vi "14.vi"(11 "n_Collatz":u64 min=1 step=1) -> (3 "max index(es)":i32)   [LabVIEW 2021]
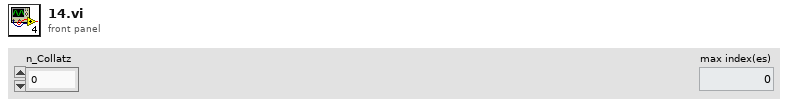
[diagram p1: front panel]
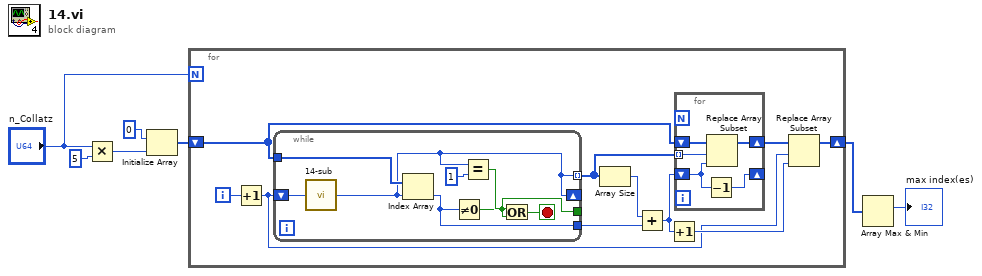
[diagram p0: block diagram]
diagram:
  n1 = Multiply(x="n_Collatz", y=u64 5) -> (x*y=w5:u64)
  n2 = Initialize Array(u64 0 ("element"), w5) -> (w6:u64[])
  n3 = for {
    N: "n_Collatz" -> [_]
    shift-right: [w16] -> w2
    shift-left: w6 -> [w17]
    i -> [w9]
    n4 = Increment(x=w9) -> (x+1=w8:i32)
    n5 = while {
      shift-right: [w27] -> _
      shift-left: w8 -> [w30]
      tunnel: [w27] -> w13 mode=indexing
      tunnel: [w24] -> w14
      tunnel: [w23] -> _
      tunnel: w17 -> [w28]
      stop <- w25 stop-if-true
      n6 = call "14-sub.vi"("n_Collatz"=w30) -> ("(n+1)_Collatz"=w27:u64)
      n7 = Index Array(array=w28, index=w27) -> (element=w24:u64)
      n8 = Not Equal To 0?(x=w24) -> (x != 0?=w23:bool)
      n9 = Equal?(x=w27, y=u64 1) -> (x = y?=w26:bool)
      n10 = Or(x=w26, y=w23) -> (x .or. y?=w25:bool)
    }
    n11 = Array Size(array=w13) -> (size(s)=w15:i32)
    n12 = Add(x=w15, y=w14) -> (x+y=w12:u64)
    n13 = Increment(x=w12) -> (x+1=w11:u64)
    n14 = for {
      tunnel: w13 -> [w20] mode=indexing
      shift-right: [w21] -> w10
      shift-left: w17 -> [w22]
      shift-right: [w18] -> _
      shift-left: w12 -> [w19]
      n15 = Decrement(x=w19) -> (x-1=w18:u64)
      n16 = Replace Array Subset(array=w22, new element=w19, index=w20) -> (w21:u64[])
    }
    n17 = Replace Array Subset(array=w10, new element=w11, index=w8) -> (w16:u64[])
  }
  n18 = Array Max & Min(array=w2) -> (max index (indices)=→"max index(es)":i32)  [unwired: 3 out]
